vi "ajustementZoneMorte.vi"(8 "Puissance Robot":dbl, 9 "Zone morte":dbl, 10 "Y":dbl, 11 "X":dbl) -> (2 "Y ajusté":dbl, 3 "X ajusté":dbl)   [LabVIEW 2019]
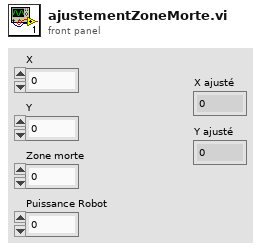
[diagram p1: front panel]
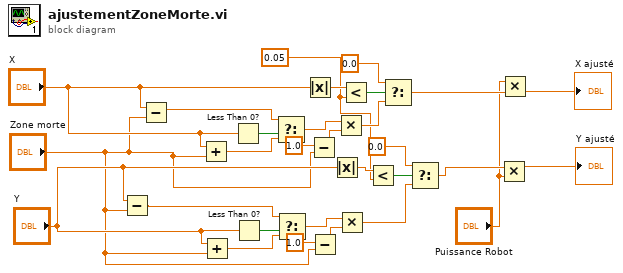
[diagram p0: block diagram]
diagram:
  w1 = 0.05
  n1 = Subtract(x="Y", y="Zone morte") -> (x-y=w8:dbl)
  n2 = Subtract(x="X", y="Zone morte") -> (x-y=w20:dbl)
  n3 = Add(x="X", y="Zone morte") -> (x+y=w18:dbl)
  n4 = Add(x="Y", y="Zone morte") -> (x+y=w10:dbl)
  n5 = Less Than 0?(x="X") -> (x < 0?=w21:bool)
  n6 = Less Than 0?(x="Y") -> (x < 0?=w9:bool)
  n7 = Select(t=w20, s=w21, f=w18) -> (s? t:f=w17:dbl)
  n8 = Select(t=w8, s=w9, f=w10) -> (s? t:f=w11:dbl)
  n9 = Absolute Value(x="X") -> (abs(x)=w28:dbl)
  n10 = Subtract(x=1.0, y="Zone morte") -> (x-y=w15:dbl)
  n11 = Subtract(x=1.0, y="Zone morte") -> (x-y=w13:dbl)
  n12 = Absolute Value(x="Y") -> (abs(x)=w24:dbl)
  n13 = Multiply(x=w17, y=w15) -> (x*y=w14:dbl)
  n14 = Multiply(x=w11, y=w13) -> (x*y=w5:dbl)
  n15 = Less?(x=w28, y=w1) -> (x < y?=w29:bool)
  n16 = Less?(x=w24, y=w1) -> (x < y?=w25:bool)
  n17 = Select(t=0.0, s=w29, f=w14) -> (s? t:f=w26:dbl)
  n18 = Select(t=0.0, s=w25, f=w5) -> (s? t:f=w22:dbl)
  n19 = Multiply(x=w22, y="Puissance Robot") -> (x*y=→"Y ajusté":dbl)
  n20 = Multiply(x="Puissance Robot", y=w26) -> (x*y=→"X ajusté":dbl)
